vi "PID_intern.vi"(6 "output range":cluster{"output high":dbl, "output low":dbl}={"output high"=100.0, "output low"=-100.0} {"output low" format="%.2f"; "output high" format="%.2f"}, 8 "dt (s)":dbl=-1.0 format="%.3f", 9 "process variable":dbl format="%.2f", 10 "setpoint":dbl format="%.2f", 11 "PID_Bitron.lvclass in":refnum<class "PID_Bitron.lvclass">) -> (0 "output":dbl format="%.2f", 3 "PID_Bitron.lvclass out":refnum<class "PID_Bitron.lvclass">)   [LabVIEW 2022 SP3, in "PID_Bitron.lvclass"]
uses:
  PID_Bitron.lvclass
  PID_Bitron.lvclass/PID_Bitron.ctl
panel:
  out "Ki*i":dbl
  out "error":dbl
  out "Kp*e":dbl
  out "Kd*d":dbl
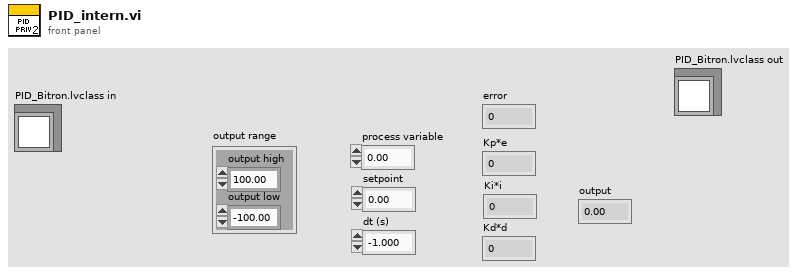
[diagram p1: front panel]
types:
  T1 = cluster{"proportional gain (Kc)":dbl, "integral time (Ti, min)":dbl, "derivative time (Td, min)":dbl}
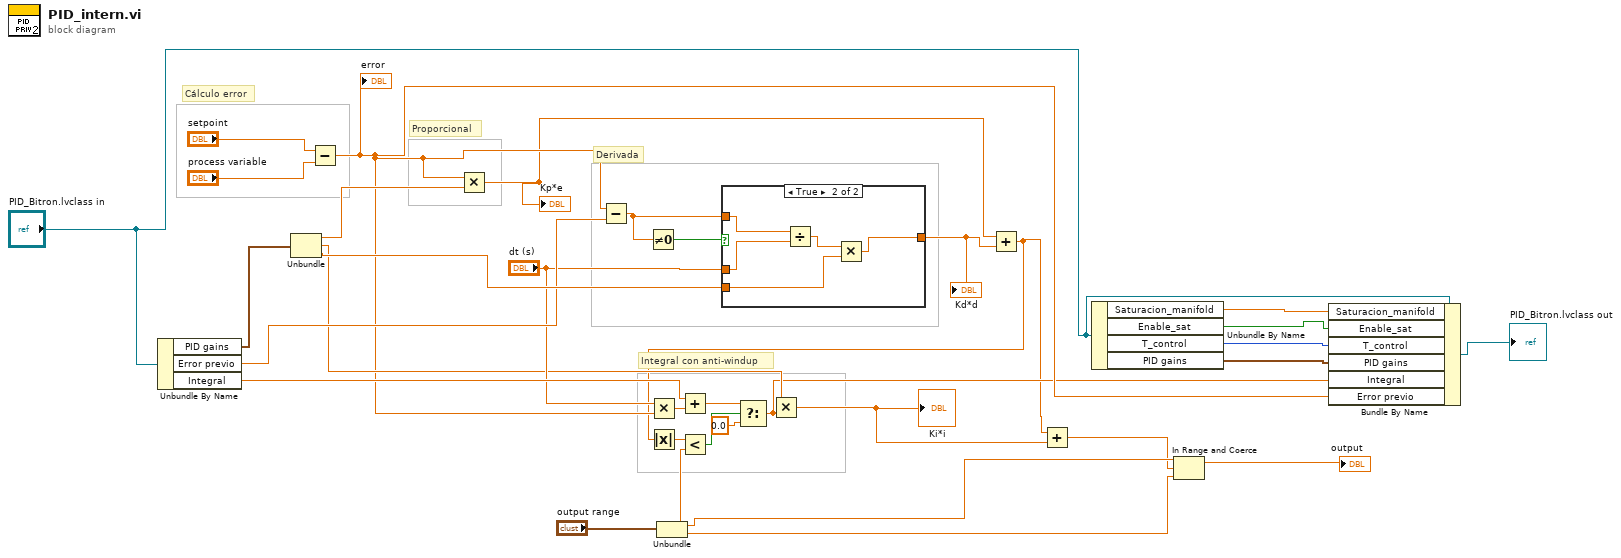
[diagram p0: block diagram]
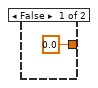
[diagram p2: hidden frame]
diagram:
  # "Integral con anti-windup"
  # "Proporcional"
  # "Cálculo error"
  # "Derivada"
  n1 = Unbundle By Name("PID_Bitron.lvclass in") -> ("PID gains"=w1:T1, "Error previo"=w22:dbl, "Integral"=w21:dbl)
  n2 = Unbundle(w1) -> ("proportional gain (Kc)"=w26:dbl, "integral time (Ti, min)"=w18:dbl, "derivative time (Td, min)"=w23:dbl)
  n3 = Subtract(x="setpoint", y="process variable") -> (x-y=w14:dbl)
  "error" <- w14
  n4 = Multiply(x=w14, y=w26) -> (x*y=w10:dbl)
  "Kp*e" <- w10
  n5 = Subtract(x=w14, y=w22) -> (x-y=w24:dbl)
  n6 = Not Equal To 0?(x=w24) -> (x != 0?=w25:bool)
  n7 = Multiply(x="dt (s)", y=w14) -> (x*y=w19:dbl)
  n8 = Unbundle("output range") -> ("output high"=w6:dbl, "output low"=w5:dbl)
  n9 = Add(x=w21, y=w19) -> (x+y=w12:dbl)
  n10 = case shown="True" w25 {
    tunnel: w24 -> [_ w39]
    tunnel: "dt (s)" -> [_ w38]
    tunnel: [0.0 w35] -> w9
    tunnel: w23 -> [_ w36]
    frame False {
    }
    frame True {
      n11 = Divide(x=w39, y=w38) -> (x/y=w37:dbl)
      n12 = Multiply(x=w37, y=w36) -> (x*y=w35:dbl)
    }
  }
  "Kd*d" <- w9
  n13 = Add(x=w10, y=w9) -> (x+y=w7:dbl)
  n14 = Absolute Value(x=w7) -> (abs(x)=w17:dbl)
  n15 = Less?(x=w17, y=w6) -> (x < y?=w16:bool)
  n16 = Select(t=w12, s=w16, f=0.0) -> (s? t:f=w11:dbl)
  n17 = Multiply(x=w18, y=w11) -> (x*y=w8:dbl)
  "Ki*i" <- w8
  n18 = Add(x=w7, y=w8) -> (x+y=w4:dbl)
  n19 = Unbundle By Name("PID_Bitron.lvclass in") -> ("Saturacion_manifold"=w30:dbl, "Enable_sat"=w29:bool, "T_control"=w28:enum16{"Manifold", "Bobina"}, "PID gains"=w27:T1)
  n20 = In Range and Coerce(upper limit=w6, x=w4, lower limit=w5) -> (coerced(x)=→"output":dbl)  [unwired: 1 out]
  n21 = Bundle By Name(cluster="PID_Bitron.lvclass in", "Saturacion_manifold"=w30, "Enable_sat"=w29, "T_control"=w28, "PID gains"=w27, "Integral"=w11, "Error previo"=w14) -> (→"PID_Bitron.lvclass out":refnum<class "PID_Bitron.lvclass">)
